vi "SIM Solve Linear Equations Triangular (single right hand).vi"(2 "matrix type":i32(ring)=1 items=["lower triangular", "upper triangular", "symmetric matrix"], 3 "Known Vector":dbl[](array[numeric]) format="%.2f", 4 "Input Matrix":T1) -> (0 "error":i32, 1 "Solution Vector":dbl[](array[numeric]) format="%.2f")   [LabVIEW 2017]
doc: "Solves a linear system AX = Y. The data types you wire to the <B>Input Matrix</B> and <B>Known Vector</B> inputs determine the polymorphic instance to use."
uses:
  RealMatrix.ctl
  <resource>/lvanlys.dll
  NI_Matrix.lvlib
panel:
  # "Solve Linear Equations"
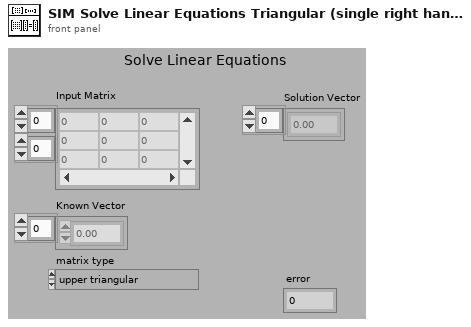
[diagram p1: front panel]
types:
  T1 = typedef "NI_Matrix.lvlib/RealMatrix.ctl" = dbl[][]
  T2 = cluster{"Compact Array":dbl[], "matrix type":i32}
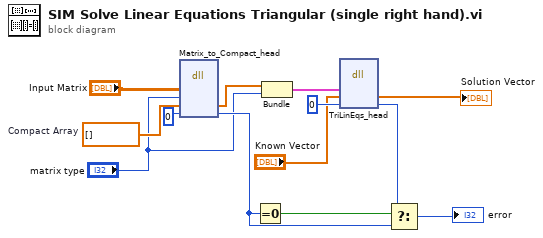
[diagram p0: block diagram]
diagram:
  w10 = dbl[] []  # Compact Array
  n1 = dll-call lib="C:/Program Files (x86)/National Instruments/LabVIEW 2017/resource/lvanlys.*" fn="Matrix_to_Compact_head" label="Real Matrix to Compact Array"("Matrix A"="Input Matrix", "matrix type"="matrix type", "Compact Array"=w10, "output param"=0) -> ("Compact Array"=w3:dbl[], "output param"=w8:i32)  [unwired: 6 in, 2 out]
  n2 = Equal To 0?(x=w8) -> (x = 0?=w12:bool)
  n3 = Bundle("Compact Array"=w3, "matrix type"="matrix type") -> (w2:T2)  [unwired: 1 in]
  n4 = dll-call lib="C:/Program Files (x86)/National Instruments/LabVIEW 2017/resource/lvanlys.*" fn="TriLinEqs_head" label="Real Compact Tri-Matrix Linear Eqs"("Triangular Compact Array"=w2, "Solution Vector"="Known Vector", "output param"=0) -> ("Solution Vector"=→"Solution Vector":dbl[], "output param"=w5:i32)  [unwired: 5 in, 2 out]
  n5 = Select(t=w5, s=w12, f=w8) -> (s? t:f=→"error":i32)
